vi "RTS MX Data.vi"(8 "Error In":errorcluster, 10 "Station":u8, 11 "Chamber 1 Data in":T1 {"Room PID Settings"."Room Dehumid Temperature I (*RM Dehum I1)" max=30000 step=1; "Room PID Settings"."Room Dehumid Temperature P (*RM Dehum P1)" max=30000 step=1; "Room PID Settings"."Room Cool Temperature I (*RM Cool I1)" max=30000 step=1; "Room PID Settings"."Room Cool Temperature P (*RM Cool P1)" max=30000 step=1; "Room PID Settings"."Room Heat I (*RM Heat I1)" max=30000 step=1; "Room PID Settings"."Room Heat P (*RM Heat P1)" max=30000 step=1; "Room PID Settings"."Room Humidity I (*RM Hum I1)" max=30000 step=1; "Room PID Settings"."Room Humidity P (*RM Hum P1)" max=30000 step=1; "Room PID Settings"."Room Dry I (*RM Dry I1)" max=30000 step=1; "Room PID Settings"."Room Dry P(*RM Dry P1)" max=30000 step=1; "Station 8"."Voltage (V):Element 1 Avg" format="%.3g"; "Station 8"."Voltage (V):Element 2 Avg" format="%.3g"; "Station 8"."Max Watt Hours" format="%.3g"; "Station 8"."Power Factor:Element 2" format="%.3g"; "Station 8"."Power Factor:Element 1" format="%.3g"; "Station 8"."Apparent Power (VA):Element 2" format="%.3g"; "Station 8"."Apparent Power (VA):Element 1" format="%.3g"; "Station 8"."Frequency (Hz):Element 1" format="%.3g"; "Station 8"."Time:Element 1" format="%.3g"; "Station 8"."Voltage Crest Factor:Element 2" format="%.3g"; "Station 8"."Voltage Crest Factor:Element 1" format="%.3g"; "Station 8"."Voltage Harmonic (%):Element 2" format="%.3g"; "Station 8"."Voltage Harmonic (%):Element 1" format="%.3g"; "Station 8"."Current Crest Factor:Element 2" format="%.3g"; "Station 8"."Current Crest Factor:Element 1" format="%.3g"; "Station 8"."Voltage (V):Element 1" format="%.3g"; "Station 8"."Voltage (V):Element 2" format="%.3g"; "Station 8"."Watt Hours (Wh):Sigma" format="%.3f"; "Station 8"."Power (W):Sigma" format="%.3g"; "Station 8"."Current (A):Element 2" format="%.3g"; "Station 8"."Current (A):Element 1" format="%.3g"; "Station 7"."Voltage (V):Element 1 Avg" format="%.3g"; "Station 7"."Voltage (V):Element 2 Avg" format="%.3g"; "Station 7"."Max Watt Hours" format="%.3g"; "Station 7"."Power Factor:Element 2" format="%.3g"; "Station 7"."Power Factor:Element 1" format="%.3g"; "Station 7"."Apparent Power (VA):Element 2" format="%.3g"; "Station 7"."Apparent Power (VA):Element 1" format="%.3g"; "Station 7"."Frequency (Hz):Element 1" format="%.3g"; "Station 7"."Time:Element 1" format="%.3g"; "Station 7"."Voltage Crest Factor:Element 2" format="%.3g"; "Station 7"."Voltage Crest Factor:Element 1" format="%.3g"; "Station 7"."Voltage Harmonic (%):Element 2" format="%.3g"; "Station 7"."Voltage Harmonic (%):Element 1" format="%.3g"; "Station 7"."Current Crest Factor:Element 2" format="%.3g"; "Station 7"."Current Crest Factor:Element 1" format="%.3g"; "Station 7"."Voltage (V):Element 1" format="%.3g"; "Station 7"."Voltage (V):Element 2" format="%.3g"; "Station 7"."Watt Hours (Wh):Sigma" format="%.3f"; "Station 7"."Power (W):Sigma" format="%.3g"; "Station 7"."Current (A):Element 2" format="%.3g"; "Station 7"."Current (A):Element 1" format="%.3g"; "Station 6"."Voltage (V):Element 1 Avg" format="%.3g"; "Station 6"."Voltage (V):Element 2 Avg" format="%.3g"; "Station 6"."Max Watt Hours" format="%.3g"; "Station 6"."Power Factor:Element 2" format="%.3g"; "Station 6"."Power Factor:Element 1" format="%.3g"; "Station 6"."Apparent Power (VA):Element 2" format="%.3g"; "Station 6"."Apparent Power (VA):Element 1" format="%.3g"; "Station 6"."Frequency (Hz):Element 1" format="%.3g"; "Station 6"."Time:Element 1" format="%.3g"; "Station 6"."Voltage Crest Factor:Element 2" format="%.3g"; "Station 6"."Voltage Crest Factor:Element 1" format="%.3g"; "Station 6"."Voltage Harmonic (%):Element 2" format="%.3g"; "Station 6"."Voltage Harmonic (%):Element 1" format="%.3g"; "Station 6"."Current Crest Factor:Element 2" format="%.3g"; "Station 6"."Current Crest Factor:Element 1" format="%.3g"; "Station 6"."Voltage (V):Element 1" format="%.3g"; "Station 6"."Voltage (V):Element 2" format="%.3g"; "Station 6"."Watt Hours (Wh):Sigma" format="%.3f"; "Station 6"."Power (W):Sigma" format="%.3g"; "Station 6"."Current (A):Element 2" format="%.3g"; "Station 6"."Current (A):Element 1" format="%.3g"; "Station 5"."Voltage (V):Element 1 Avg" format="%.3g"; "Station 5"."Voltage (V):Element 2 Avg" format="%.3g"; "Station 5"."Max Watt Hours" format="%.3g"; "Station 5"."Power Factor:Element 2" format="%.3g"; "Station 5"."Power Factor:Element 1" format="%.3g"; "Station 5"."Apparent Power (VA):Element 2" format="%.3g"; "Station 5"."Apparent Power (VA):Element 1" format="%.3g"; "Station 5"."Frequency (Hz):Element 1" format="%.3g"; "Station 5"."Time:Element 1" format="%.3g"; "Station 5"."Voltage Crest Factor:Element 2" format="%.3g"; "Station 5"."Voltage Crest Factor:Element 1" format="%.3g"; "Station 5"."Voltage Harmonic (%):Element 2" format="%.3g"; "Station 5"."Voltage Harmonic (%):Element 1" format="%.3g"; "Station 5"."Current Crest Factor:Element 2" format="%.3g"; "Station 5"."Current Crest Factor:Element 1" format="%.3g"; "Station 5"."Voltage (V):Element 1" format="%.3g"; "Station 5"."Voltage (V):Element 2" format="%.3g"; "Station 5"."Watt Hours (Wh):Sigma" format="%.3f"; "Station 5"."Power (W):Sigma" format="%.3g"; "Station 5"."Current (A):Element 2" format="%.3g"; "Station 5"."Current (A):Element 1" format="%.3g"; "Station 4"."Voltage (V):Element 1 Avg" format="%.3g"; "Station 4"."Voltage (V):Element 2 Avg" format="%.3g"; "Station 4"."Max Watt Hours" format="%.3g"; "Station 4"."Power Factor:Element 2" format="%.3g"; "Station 4"."Power Factor:Element 1" format="%.3g"; "Station 4"."Apparent Power (VA):Element 2" format="%.3g"; "Station 4"."Apparent Power (VA):Element 1" format="%.3g"; "Station 4"."Frequency (Hz):Element 1" format="%.3g"; "Station 4"."Time:Element 1" format="%.3g"; "Station 4"."Voltage Crest Factor:Element 2" format="%.3g"; "Station 4"."Voltage Crest Factor:Element 1" format="%.3g"; "Station 4"."Voltage Harmonic (%):Element 2" format="%.3g"; "Station 4"."Voltage Harmonic (%):Element 1" format="%.3g"; "Station 4"."Current Crest Factor:Element 2" format="%.3g"; "Station 4"."Current Crest Factor:Element 1" format="%.3g"; "Station 4"."Voltage (V):Element 1" format="%.3g"; "Station 4"."Voltage (V):Element 2" format="%.3g"; "Station 4"."Watt Hours (Wh):Sigma" format="%.3f"; "Station 4"."Power (W):Sigma" format="%.3g"; "Station 4"."Current (A):Element 2" format="%.3g"; "Station 4"."Current (A):Element 1" format="%.3g"; "Station 3"."Voltage (V):Element 1 Avg" format="%.3g"; "Station 3"."Voltage (V):Element 2 Avg" format="%.3g"; "Station 3"."Max Watt Hours" format="%.3g"; "Station 3"."Power Factor:Element 2" format="%.3g"; "Station 3"."Power Factor:Element 1" format="%.3g"; "Station 3"."Apparent Power (VA):Element 2" format="%.3g"; "Station 3"."Apparent Power (VA):Element 1" format="%.3g"; "Station 3"."Frequency (Hz):Element 1" format="%.3g"; "Station 3"."Time:Element 1" format="%.3g"; "Station 3"."Voltage Crest Factor:Element 2" format="%.3g"; "Station 3"."Voltage Crest Factor:Element 1" format="%.3g"; "Station 3"."Voltage Harmonic (%):Element 2" format="%.3g"; "Station 3"."Voltage Harmonic (%):Element 1" format="%.3g"; "Station 3"."Current Crest Factor:Element 2" format="%.3g"; "Station 3"."Current Crest Factor:Element 1" format="%.3g"; "Station 3"."Voltage (V):Element 1" format="%.3g"; "Station 3"."Voltage (V):Element 2" format="%.3g"; "Station 3"."Watt Hours (Wh):Sigma" format="%.3f"; "Station 3"."Power (W):Sigma" format="%.3g"; "Station 3"."Current (A):Element 2" format="%.3g"; "Station 3"."Current (A):Element 1" format="%.3g"; "Station 2"."Voltage (V):Element 1 Avg" format="%.3g"; "Station 2"."Voltage (V):Element 2 Avg" format="%.3g"; "Station 2"."Max Watt Hours" format="%.3g"; "Station 2"."Power Factor:Element 2" format="%.3g"; "Station 2"."Power Factor:Element 1" format="%.3g"; "Station 2"."Apparent Power (VA):Element 2" format="%.3g"; "Station 2"."Apparent Power (VA):Element 1" format="%.3g"; "Station 2"."Frequency (Hz):Element 1" format="%.3g"; "Station 2"."Time:Element 1" format="%.3g"; "Station 2"."Voltage Crest Factor:Element 2" format="%.3g"; "Station 2"."Voltage Crest Factor:Element 1" format="%.3g"; "Station 2"."Voltage Harmonic (%):Element 2" format="%.3g"; "Station 2"."Voltage Harmonic (%):Element 1" format="%.3g"; "Station 2"."Current Crest Factor:Element 2" format="%.3g"; "Station 2"."Current Crest Factor:Element 1" format="%.3g"; "Station 2"."Voltage (V):Element 1" format="%.3g"; "Station 2"."Voltage (V):Element 2" format="%.3g"; "Station 2"."Watt Hours (Wh):Sigma" format="%.3f"; "Station 2"."Power (W):Sigma" format="%.3g"; "Station 2"."Current (A):Element 2" format="%.3g"; "Station 2"."Current (A):Element 1" format="%.3g"; "Station 1"."Voltage (V):Element 1 Avg" format="%.3g"; "Station 1"."Voltage (V):Element 2 Avg" format="%.3g"; "Station 1"."Max Watt Hours" format="%.3g"; "Station 1"."Power Factor:Element 2" format="%.3g"; "Station 1"."Power Factor:Element 1" format="%.3g"; "Station 1"."Apparent Power (VA):Element 2" format="%.3g"; "Station 1"."Apparent Power (VA):Element 1" format="%.3g"; "Station 1"."Frequency (Hz):Element 1" format="%.3g"; "Station 1"."Time:Element 1" format="%.3g"; "Station 1"."Voltage Crest Factor:Element 2" format="%.3g"; "Station 1"."Voltage Crest Factor:Element 1" format="%.3g"; "Station 1"."Voltage Harmonic (%):Element 2" format="%.3g"; "Station 1"."Voltage Harmonic (%):Element 1" format="%.3g"; "Station 1"."Current Crest Factor:Element 2" format="%.3g"; "Station 1"."Current Crest Factor:Element 1" format="%.3g"; "Station 1"."Voltage (V):Element 1" format="%.3g"; "Station 1"."Voltage (V):Element 2" format="%.3g"; "Station 1"."Watt Hours (Wh):Sigma" format="%.3f"; "Station 1"."Power (W):Sigma" format="%.3g"; "Station 1"."Current (A):Element 2" format="%.3g"; "Station 1"."Current (A):Element 1" format="%.3g"}) -> (0 "Error Out":errorcluster, 1 "Data MX (DBL)":dbl[](array[numeric]), 2 "Data MX":string[][](array[string]), 3 "Chamber 1 Data Out":T1 {"Room PID Settings"."Room Dehumid Temperature I (*RM Dehum I1)" max=30000 step=1; "Room PID Settings"."Room Dehumid Temperature P (*RM Dehum P1)" max=30000 step=1; "Room PID Settings"."Room Cool Temperature I (*RM Cool I1)" max=30000 step=1; "Room PID Settings"."Room Cool Temperature P (*RM Cool P1)" max=30000 step=1; "Room PID Settings"."Room Heat I (*RM Heat I1)" max=30000 step=1; "Room PID Settings"."Room Heat P (*RM Heat P1)" max=30000 step=1; "Room PID Settings"."Room Humidity I (*RM Hum I1)" max=30000 step=1; "Room PID Settings"."Room Humidity P (*RM Hum P1)" max=30000 step=1; "Room PID Settings"."Room Dry I (*RM Dry I1)" max=30000 step=1; "Room PID Settings"."Room Dry P(*RM Dry P1)" max=30000 step=1; "Station 8"."Voltage (V):Element 1 Avg" format="%.3g"; "Station 8"."Voltage (V):Element 2 Avg" format="%.3g"; "Station 8"."Max Watt Hours" format="%.3g"; "Station 8"."Power Factor:Element 2" format="%.3g"; "Station 8"."Power Factor:Element 1" format="%.3g"; "Station 8"."Apparent Power (VA):Element 2" format="%.3g"; "Station 8"."Apparent Power (VA):Element 1" format="%.3g"; "Station 8"."Frequency (Hz):Element 1" format="%.3g"; "Station 8"."Time:Element 1" format="%.3g"; "Station 8"."Voltage Crest Factor:Element 2" format="%.3g"; "Station 8"."Voltage Crest Factor:Element 1" format="%.3g"; "Station 8"."Voltage Harmonic (%):Element 2" format="%.3g"; "Station 8"."Voltage Harmonic (%):Element 1" format="%.3g"; "Station 8"."Current Crest Factor:Element 2" format="%.3g"; "Station 8"."Current Crest Factor:Element 1" format="%.3g"; "Station 8"."Voltage (V):Element 1" format="%.3g"; "Station 8"."Voltage (V):Element 2" format="%.3g"; "Station 8"."Watt Hours (Wh):Sigma" format="%.3f"; "Station 8"."Power (W):Sigma" format="%.3g"; "Station 8"."Current (A):Element 2" format="%.3g"; "Station 8"."Current (A):Element 1" format="%.3g"; "Station 7"."Voltage (V):Element 1 Avg" format="%.3g"; "Station 7"."Voltage (V):Element 2 Avg" format="%.3g"; "Station 7"."Max Watt Hours" format="%.3g"; "Station 7"."Power Factor:Element 2" format="%.3g"; "Station 7"."Power Factor:Element 1" format="%.3g"; "Station 7"."Apparent Power (VA):Element 2" format="%.3g"; "Station 7"."Apparent Power (VA):Element 1" format="%.3g"; "Station 7"."Frequency (Hz):Element 1" format="%.3g"; "Station 7"."Time:Element 1" format="%.3g"; "Station 7"."Voltage Crest Factor:Element 2" format="%.3g"; "Station 7"."Voltage Crest Factor:Element 1" format="%.3g"; "Station 7"."Voltage Harmonic (%):Element 2" format="%.3g"; "Station 7"."Voltage Harmonic (%):Element 1" format="%.3g"; "Station 7"."Current Crest Factor:Element 2" format="%.3g"; "Station 7"."Current Crest Factor:Element 1" format="%.3g"; "Station 7"."Voltage (V):Element 1" format="%.3g"; "Station 7"."Voltage (V):Element 2" format="%.3g"; "Station 7"."Watt Hours (Wh):Sigma" format="%.3f"; "Station 7"."Power (W):Sigma" format="%.3g"; "Station 7"."Current (A):Element 2" format="%.3g"; "Station 7"."Current (A):Element 1" format="%.3g"; "Station 6"."Voltage (V):Element 1 Avg" format="%.3g"; "Station 6"."Voltage (V):Element 2 Avg" format="%.3g"; "Station 6"."Max Watt Hours" format="%.3g"; "Station 6"."Power Factor:Element 2" format="%.3g"; "Station 6"."Power Factor:Element 1" format="%.3g"; "Station 6"."Apparent Power (VA):Element 2" format="%.3g"; "Station 6"."Apparent Power (VA):Element 1" format="%.3g"; "Station 6"."Frequency (Hz):Element 1" format="%.3g"; "Station 6"."Time:Element 1" format="%.3g"; "Station 6"."Voltage Crest Factor:Element 2" format="%.3g"; "Station 6"."Voltage Crest Factor:Element 1" format="%.3g"; "Station 6"."Voltage Harmonic (%):Element 2" format="%.3g"; "Station 6"."Voltage Harmonic (%):Element 1" format="%.3g"; "Station 6"."Current Crest Factor:Element 2" format="%.3g"; "Station 6"."Current Crest Factor:Element 1" format="%.3g"; "Station 6"."Voltage (V):Element 1" format="%.3g"; "Station 6"."Voltage (V):Element 2" format="%.3g"; "Station 6"."Watt Hours (Wh):Sigma" format="%.3f"; "Station 6"."Power (W):Sigma" format="%.3g"; "Station 6"."Current (A):Element 2" format="%.3g"; "Station 6"."Current (A):Element 1" format="%.3g"; "Station 5"."Voltage (V):Element 1 Avg" format="%.3g"; "Station 5"."Voltage (V):Element 2 Avg" format="%.3g"; "Station 5"."Max Watt Hours" format="%.3g"; "Station 5"."Power Factor:Element 2" format="%.3g"; "Station 5"."Power Factor:Element 1" format="%.3g"; "Station 5"."Apparent Power (VA):Element 2" format="%.3g"; "Station 5"."Apparent Power (VA):Element 1" format="%.3g"; "Station 5"."Frequency (Hz):Element 1" format="%.3g"; "Station 5"."Time:Element 1" format="%.3g"; "Station 5"."Voltage Crest Factor:Element 2" format="%.3g"; "Station 5"."Voltage Crest Factor:Element 1" format="%.3g"; "Station 5"."Voltage Harmonic (%):Element 2" format="%.3g"; "Station 5"."Voltage Harmonic (%):Element 1" format="%.3g"; "Station 5"."Current Crest Factor:Element 2" format="%.3g"; "Station 5"."Current Crest Factor:Element 1" format="%.3g"; "Station 5"."Voltage (V):Element 1" format="%.3g"; "Station 5"."Voltage (V):Element 2" format="%.3g"; "Station 5"."Watt Hours (Wh):Sigma" format="%.3f"; "Station 5"."Power (W):Sigma" format="%.3g"; "Station 5"."Current (A):Element 2" format="%.3g"; "Station 5"."Current (A):Element 1" format="%.3g"; "Station 4"."Voltage (V):Element 1 Avg" format="%.3g"; "Station 4"."Voltage (V):Element 2 Avg" format="%.3g"; "Station 4"."Max Watt Hours" format="%.3g"; "Station 4"."Power Factor:Element 2" format="%.3g"; "Station 4"."Power Factor:Element 1" format="%.3g"; "Station 4"."Apparent Power (VA):Element 2" format="%.3g"; "Station 4"."Apparent Power (VA):Element 1" format="%.3g"; "Station 4"."Frequency (Hz):Element 1" format="%.3g"; "Station 4"."Time:Element 1" format="%.3g"; "Station 4"."Voltage Crest Factor:Element 2" format="%.3g"; "Station 4"."Voltage Crest Factor:Element 1" format="%.3g"; "Station 4"."Voltage Harmonic (%):Element 2" format="%.3g"; "Station 4"."Voltage Harmonic (%):Element 1" format="%.3g"; "Station 4"."Current Crest Factor:Element 2" format="%.3g"; "Station 4"."Current Crest Factor:Element 1" format="%.3g"; "Station 4"."Voltage (V):Element 1" format="%.3g"; "Station 4"."Voltage (V):Element 2" format="%.3g"; "Station 4"."Watt Hours (Wh):Sigma" format="%.3f"; "Station 4"."Power (W):Sigma" format="%.3g"; "Station 4"."Current (A):Element 2" format="%.3g"; "Station 4"."Current (A):Element 1" format="%.3g"; "Station 3"."Voltage (V):Element 1 Avg" format="%.3g"; "Station 3"."Voltage (V):Element 2 Avg" format="%.3g"; "Station 3"."Max Watt Hours" format="%.3g"; "Station 3"."Power Factor:Element 2" format="%.3g"; "Station 3"."Power Factor:Element 1" format="%.3g"; "Station 3"."Apparent Power (VA):Element 2" format="%.3g"; "Station 3"."Apparent Power (VA):Element 1" format="%.3g"; "Station 3"."Frequency (Hz):Element 1" format="%.3g"; "Station 3"."Time:Element 1" format="%.3g"; "Station 3"."Voltage Crest Factor:Element 2" format="%.3g"; "Station 3"."Voltage Crest Factor:Element 1" format="%.3g"; "Station 3"."Voltage Harmonic (%):Element 2" format="%.3g"; "Station 3"."Voltage Harmonic (%):Element 1" format="%.3g"; "Station 3"."Current Crest Factor:Element 2" format="%.3g"; "Station 3"."Current Crest Factor:Element 1" format="%.3g"; "Station 3"."Voltage (V):Element 1" format="%.3g"; "Station 3"."Voltage (V):Element 2" format="%.3g"; "Station 3"."Watt Hours (Wh):Sigma" format="%.3f"; "Station 3"."Power (W):Sigma" format="%.3g"; "Station 3"."Current (A):Element 2" format="%.3g"; "Station 3"."Current (A):Element 1" format="%.3g"; "Station 2"."Voltage (V):Element 1 Avg" format="%.3g"; "Station 2"."Voltage (V):Element 2 Avg" format="%.3g"; "Station 2"."Max Watt Hours" format="%.3g"; "Station 2"."Power Factor:Element 2" format="%.3g"; "Station 2"."Power Factor:Element 1" format="%.3g"; "Station 2"."Apparent Power (VA):Element 2" format="%.3g"; "Station 2"."Apparent Power (VA):Element 1" format="%.3g"; "Station 2"."Frequency (Hz):Element 1" format="%.3g"; "Station 2"."Time:Element 1" format="%.3g"; "Station 2"."Voltage Crest Factor:Element 2" format="%.3g"; "Station 2"."Voltage Crest Factor:Element 1" format="%.3g"; "Station 2"."Voltage Harmonic (%):Element 2" format="%.3g"; "Station 2"."Voltage Harmonic (%):Element 1" format="%.3g"; "Station 2"."Current Crest Factor:Element 2" format="%.3g"; "Station 2"."Current Crest Factor:Element 1" format="%.3g"; "Station 2"."Voltage (V):Element 1" format="%.3g"; "Station 2"."Voltage (V):Element 2" format="%.3g"; "Station 2"."Watt Hours (Wh):Sigma" format="%.3f"; "Station 2"."Power (W):Sigma" format="%.3g"; "Station 2"."Current (A):Element 2" format="%.3g"; "Station 2"."Current (A):Element 1" format="%.3g"; "Station 1"."Voltage (V):Element 1 Avg" format="%.3g"; "Station 1"."Voltage (V):Element 2 Avg" format="%.3g"; "Station 1"."Max Watt Hours" format="%.3g"; "Station 1"."Power Factor:Element 2" format="%.3g"; "Station 1"."Power Factor:Element 1" format="%.3g"; "Station 1"."Apparent Power (VA):Element 2" format="%.3g"; "Station 1"."Apparent Power (VA):Element 1" format="%.3g"; "Station 1"."Frequency (Hz):Element 1" format="%.3g"; "Station 1"."Time:Element 1" format="%.3g"; "Station 1"."Voltage Crest Factor:Element 2" format="%.3g"; "Station 1"."Voltage Crest Factor:Element 1" format="%.3g"; "Station 1"."Voltage Harmonic (%):Element 2" format="%.3g"; "Station 1"."Voltage Harmonic (%):Element 1" format="%.3g"; "Station 1"."Current Crest Factor:Element 2" format="%.3g"; "Station 1"."Current Crest Factor:Element 1" format="%.3g"; "Station 1"."Voltage (V):Element 1" format="%.3g"; "Station 1"."Voltage (V):Element 2" format="%.3g"; "Station 1"."Watt Hours (Wh):Sigma" format="%.3f"; "Station 1"."Power (W):Sigma" format="%.3g"; "Station 1"."Current (A):Element 2" format="%.3g"; "Station 1"."Current (A):Element 1" format="%.3g"})   [LabVIEW 2016]
uses:
  Type Definitions/RTS Chamber Data.ctl
  Utility/Type Definitions/UTILITY Power Data.ctl
  Type Definitions/RTS Chamber TCs.ctl
  Type Definitions/RTS MX5 AUX Data.ctl
  Drivers/WAGO 750-881/Type Definitions/Wago Door Relays.ctl
  Drivers/WAGO 750-881/Type Definitions/Wago Contactor Settings.ctl
  Drivers/WAGO 750-881/Type Definitions/Wago Ground Leakage.ctl
  Drivers/WAGO 750-881/Type Definitions/Wago Measured Input Data.ctl
  Drivers/WAGO 750-881/Type Definitions/Wago Room Setpoint Targets.ctl
  Drivers/WAGO 750-881/Type Definitions/Wago Room PID Settings.ctl
  Drivers/WAGO 750-881/Type Definitions/Wago Room Condtions.ctl
panel:
  # "APLUS"
  # "MX100"
  # "Wago Controller"
  # "APLUS"
  # "MX100"
  # "Wago Controller"
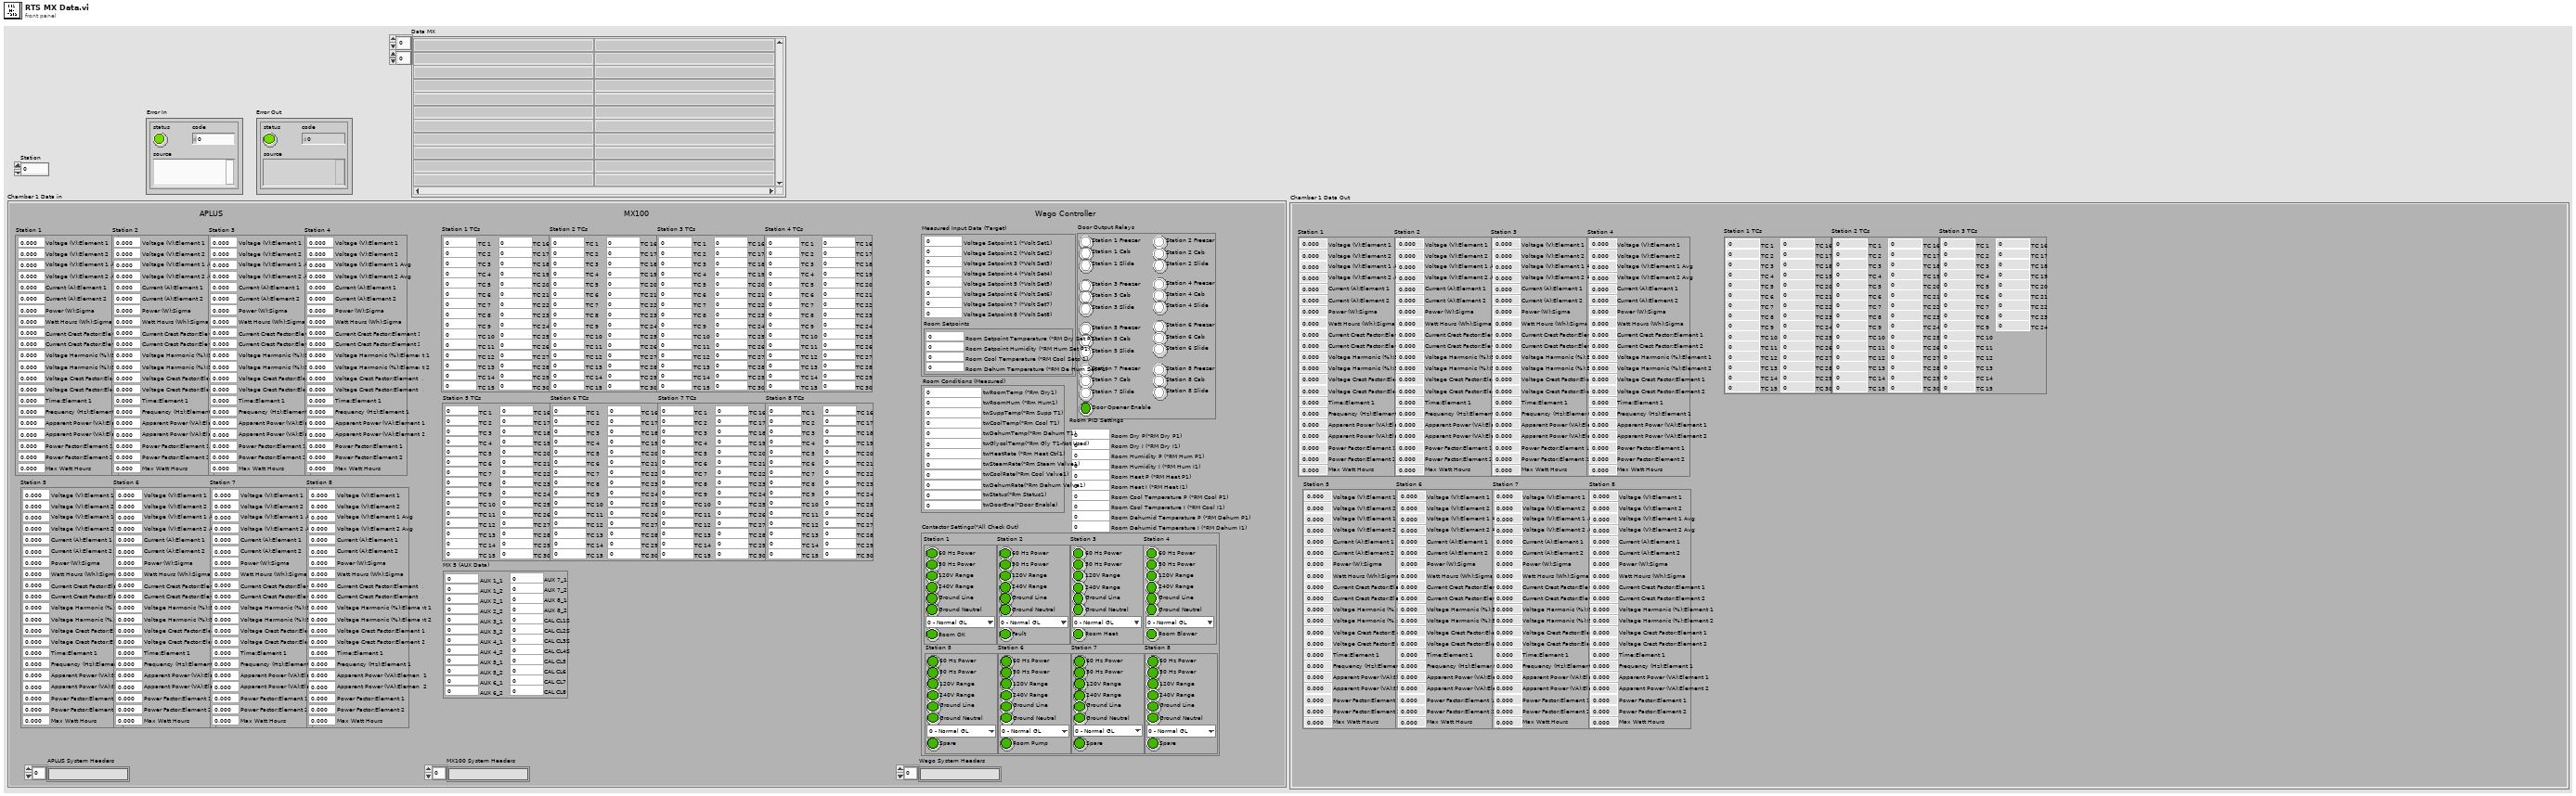
[diagram p1: front panel]
types:
  T1 = typedef "RTS Chamber Data.ctl" = cluster{"Station 1":T2, "Station 2":T2, "Station 3":T2, "Station 4":T2, "Station 5":T2, "Station 6":T2, "Station 7":T2, "Station 8":T2, "Station 1 TCs":T3, "Station 2 TCs":T3, "Station 3 TCs":T3, "Station 4 TCs":T3, "Station 5 TCs":T3, "Station 6 TCs":T3, "Station 7 TCs":T3, "Station 8 TCs":T3, "MX 5 (AUX Data)":T4, "Door Output Relays":T5, "Contactor Settings(*All Check Out)":T6, "Measured Input Data (Target)":T8, "Room PID Settings":T10, "Room Conditions (Measured)":T11, "APLUS System Headers":string[], "MX100 System Headers":string[], "Wago System Headers":string[]}
  T2 = typedef "UTILITY Power Data.ctl" = cluster{"Current (A):Element 1":dbl, "Current (A):Element 2":dbl, "Power (W):Sigma":dbl, "Watt Hours (Wh):Sigma":dbl, "Voltage (V):Element 2":dbl, "Voltage (V):Element 1":dbl, "Current Crest Factor:Element 1":dbl, "Current Crest Factor:Element 2":dbl, "Voltage Harmonic (%):Element 1":dbl, "Voltage Harmonic (%):Element 2":dbl, "Voltage Crest Factor:Element 1":dbl, "Voltage Crest Factor:Element 2":dbl, "Time:Element 1":dbl, "Frequency (Hz):Element 1":dbl, "Apparent Power (VA):Element 1":dbl, "Apparent Power (VA):Element 2":dbl, "Power Factor:Element 1":dbl, "Power Factor:Element 2":dbl, "Max Watt Hours":dbl, "Voltage (V):Element 2 Avg":dbl, "Voltage (V):Element 1 Avg":dbl}
  T3 = typedef "RTS Chamber TCs.ctl" = cluster{"TC 1":dbl, "TC 2":dbl, "TC 3":dbl, "TC 4":dbl, "TC 5":dbl, "TC 6":dbl, "TC 7":dbl, "TC 8":dbl, "TC 9":dbl, "TC 10":dbl, "TC 11":dbl, "TC 12":dbl, "TC 13":dbl, "TC 14":dbl, "TC 15":dbl, "TC 16":dbl, "TC 17":dbl, "TC 18":dbl, "TC 19":dbl, "TC 20":dbl, "TC 21":dbl, "TC 22":dbl, "TC 23":dbl, "TC 24":dbl, "TC 25":dbl, "TC 26":dbl, "TC 27":dbl, "TC 28":dbl, "TC 29":dbl, "TC 30":dbl}
  T4 = typedef "RTS MX5 AUX Data.ctl" = cluster{"AUX 1_1":dbl, "AUX 1_2":dbl, "AUX 2_1":dbl, "AUX 2_2":dbl, "AUX 3_1":dbl, "AUX 3_2":dbl, "AUX 4_1":dbl, "AUX 4_2":dbl, "AUX 5_1":dbl, "AUX 5_2":dbl, "AUX 6_1":dbl, "AUX 6_2":dbl, "AUX 7_1":dbl, "AUX 7_2":dbl, "AUX 8_1":dbl, "AUX 8_2":dbl, "CAL CL1S":dbl, "CAL CL2S":dbl, "CAL CL3S":dbl, "CAL CL4S":dbl, "CAL CL5":dbl, "CAL CL6":dbl, "CAL CL7":dbl, "CAL CL8":dbl}
  T5 = typedef "Wago Door Relays.ctl" = cluster{"Station 1 Freezer":bool, "Station 1 Cab":bool, "Station 1 Slide":bool, "Station 2 Freezer":bool, "Station 2 Cab":bool, "Station 2 Slide":bool, "Station 3 Freezer":bool, "Station 3 Cab":bool, "Station 3 Slide":bool, "Station 4 Freezer":bool, "Station 4 Cab":bool, "Station 4 Slide":bool, "Station 5 Freezer":bool, "Station 5 Cab":bool, "Station 5 Slide":bool, "Station 6 Freezer":bool, "Station 6 Cab":bool, "Station 6 Slide":bool, "Station 7 Freezer":bool, "Station 7 Cab":bool, "Station 7 Slide":bool, "Station 8 Freezer":bool, "Station 8 Cab":bool, "Station 8 Slide":bool, "Door Opener Enable":bool}
  T6 = typedef "Wago Contactor Settings.ctl" = cluster{"Station 1":cluster{"60 Hz Power":bool, "50 Hz Power":bool, "120V Range":bool, "240V Range":bool, "Ground Line":bool, "Ground Neutral":bool, "Room OK":bool, "Ground Leakage":T7}, "Station 2":cluster{"60 Hz Power":bool, "50 Hz Power":bool, "120V Range":bool, "240V Range":bool, "Ground Line":bool, "Ground Neutral":bool, "Fault":bool, "Ground Leakage":T7}, "Station 3":cluster{"60 Hz Power":bool, "50 Hz Power":bool, "120V Range":bool, "240V Range":bool, "Ground Line":bool, "Ground Neutral":bool, "Room Heat":bool, "Ground Leakage":T7}, "Station 4":cluster{"60 Hz Power":bool, "50 Hz Power":bool, "120V Range":bool, "240V Range":bool, "Ground Line":bool, "Ground Neutral":bool, "Room Blower":bool, "Ground Leakage":T7}, "Station 5":cluster{"60 Hz Power":bool, "50 Hz Power":bool, "120V Range":bool, "240V Range":bool, "Ground Line":bool, "Ground Neutral":bool, "Spare":bool, "Ground Leakage":T7}, "Station 6":cluster{"60 Hz Power":bool, "50 Hz Power":bool, "120V Range":bool, "240V Range":bool, "Ground Line":bool, "Ground Neutral":bool, "Room Pump":bool, "Ground Leakage":T7}, "Station 7":cluster{"60 Hz Power":bool, "50 Hz Power":bool, "120V Range":bool, "240V Range":bool, "Ground Line":bool, "Ground Neutral":bool, "Spare":bool, "Ground Leakage":T7}, "Station 8":cluster{"60 Hz Power":bool, "50 Hz Power":bool, "120V Range":bool, "240V Range":bool, "Ground Line":bool, "Ground Neutral":bool, "Spare":bool, "Ground Leakage":T7}}
  T7 = typedef "Wago Ground Leakage.ctl" = enum16{"0 - Normal GL", "1 - Measure GL"}
  T8 = typedef "Wago Measured Input Data.ctl" = cluster{"Voltage Setpoint 1 (*Volt Set1)":dbl, "Voltage Setpoint 2 (*Volt Set2)":dbl, "Voltage Setpoint 3 (*Volt Set3)":dbl, "Voltage Setpoint 4 (*Volt Set4)":dbl, "Voltage Setpoint 5 (*Volt Set5)":dbl, "Voltage Setpoint 6 (*Volt Set6)":dbl, "Voltage Setpoint 7 (*Volt Set7)":dbl, "Voltage Setpoint 8 (*Volt Set8)":dbl, "Room Setpoints":T9}
  T9 = typedef "Wago Room Setpoint Targets.ctl" = cluster{"Room Setpoint Temperature (*RM Dry Set P1)":dbl, "Room Setpoint Humidity (*RM Hum Set P1)":dbl, "Room Cool Temperature (*RM Cool Setp 1)":dbl, "Room Dehum Temperature (*RM De Hum Set P1)":dbl}
  T10 = typedef "Wago Room PID Settings.ctl" = cluster{"Room Dry P(*RM Dry P1)":u16, "Room Dry I (*RM Dry I1)":u16, "Room Humidity P (*RM Hum P1)":u16, "Room Humidity I (*RM Hum I1)":u16, "Room Heat P (*RM Heat P1)":u16, "Room Heat I (*RM Heat I1)":u16, "Room Cool Temperature P (*RM Cool P1)":u16, "Room Cool Temperature I (*RM Cool I1)":u16, "Room Dehumid Temperature P (*RM Dehum P1)":u16, "Room Dehumid Temperature I (*RM Dehum I1)":u16}
  T11 = typedef "Wago Room Condtions.ctl" = cluster{"twDoorEna(*Door Enable)":u16, "twStatus(*Rm Status1)":u16, "twRoomTemp (*Rm Dry1)":dbl, "twRoomHum (*Rm Hum1)":dbl, "twSuppTemp(*Rm Supp T1)":dbl, "twCoolTemp(*Rm Cool T1)":dbl, "twDehumTemp(*Rm Dehum T1)":dbl, "twGlycolTemp(*Rm Gly T1-Not Used)":dbl, "twDehumRate(*Rm Dehum Valve1)":dbl, "twCoolRate(*Rm Cool Valve1)":dbl, "twSteamRate(*Rm Steam Valve1)":dbl, "twHeatRate (*Rm Heat Ctrl1)":dbl}
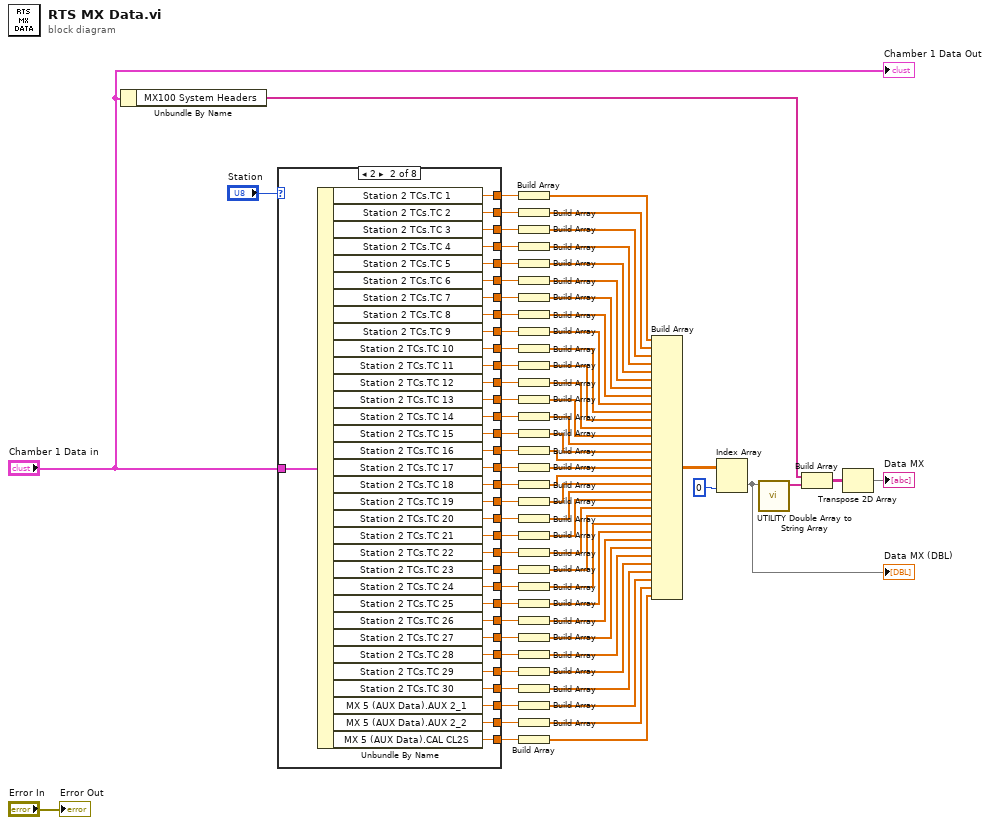
[diagram p0: block diagram]
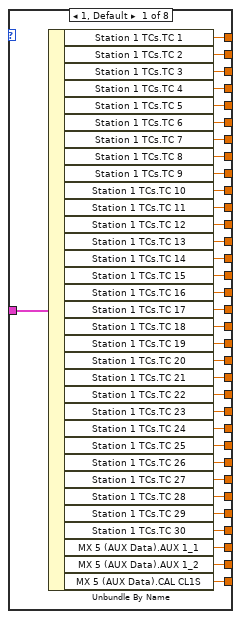
[diagram p2: hidden frame]
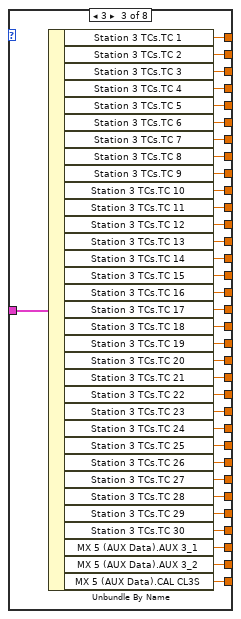
[diagram p3: hidden frame]
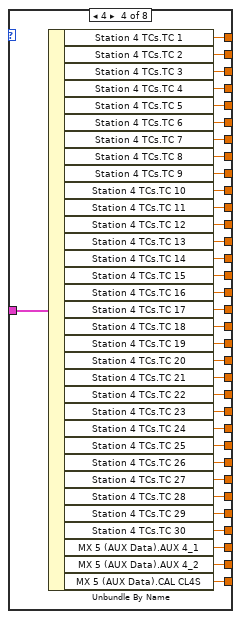
[diagram p4: hidden frame]
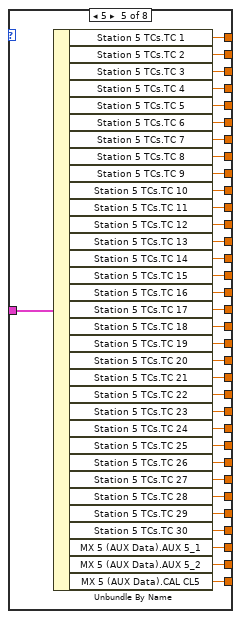
[diagram p5: hidden frame]
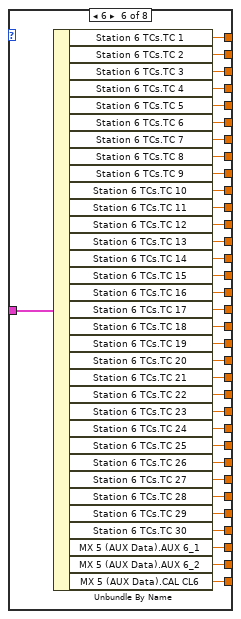
[diagram p6: hidden frame]
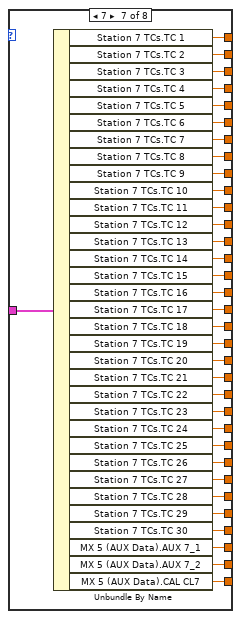
[diagram p7: hidden frame]
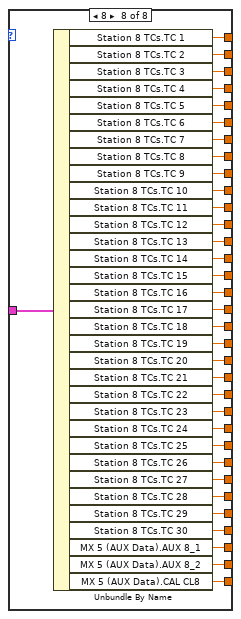
[diagram p8: hidden frame]
diagram:
  n1 = Unbundle By Name("Chamber 1 Data in") -> ("MX100 System Headers"=w38:string[])
  n2 = case shown="2" "Station" {
    tunnel: "Chamber 1 Data in" -> [w110 w144 w178 w212 w246 w280 w314 w348]
    tunnel: [w109 w143 w177 w211 w245 w279 w313 w347] -> w44
    tunnel: [w108 w142 w176 w210 w244 w278 w312 w346] -> w45
    tunnel: [w107 w141 w175 w209 w243 w277 w311 w345] -> w46
    tunnel: [w106 w140 w174 w208 w242 w276 w310 w344] -> w47
    tunnel: [w105 w139 w173 w207 w241 w275 w309 w343] -> w48
    tunnel: [w104 w138 w172 w206 w240 w274 w308 w342] -> w49
    tunnel: [w103 w137 w171 w205 w239 w273 w307 w341] -> w50
    tunnel: [w102 w136 w170 w204 w238 w272 w306 w340] -> w51
    tunnel: [w101 w135 w169 w203 w237 w271 w305 w339] -> w52
    tunnel: [w100 w134 w168 w202 w236 w270 w304 w338] -> w53
    tunnel: [w99 w133 w167 w201 w235 w269 w303 w337] -> w54
    tunnel: [w98 w132 w166 w200 w234 w268 w302 w336] -> w55
    tunnel: [w97 w131 w165 w199 w233 w267 w301 w335] -> w56
    tunnel: [w96 w130 w164 w198 w232 w266 w300 w334] -> w57
    tunnel: [w95 w129 w163 w197 w231 w265 w299 w333] -> w58
    tunnel: [w94 w128 w162 w196 w230 w264 w298 w332] -> w59
    tunnel: [w93 w127 w161 w195 w229 w263 w297 w331] -> w60
    tunnel: [w92 w126 w160 w194 w228 w262 w296 w330] -> w61
    tunnel: [w91 w125 w159 w193 w227 w261 w295 w329] -> w62
    tunnel: [w90 w124 w158 w192 w226 w260 w294 w328] -> w63
    tunnel: [w89 w123 w157 w191 w225 w259 w293 w327] -> w64
    tunnel: [w88 w122 w156 w190 w224 w258 w292 w326] -> w65
    tunnel: [w87 w121 w155 w189 w223 w257 w291 w325] -> w66
    tunnel: [w86 w120 w154 w188 w222 w256 w290 w324] -> w67
    tunnel: [w85 w119 w153 w187 w221 w255 w289 w323] -> w68
    tunnel: [w84 w118 w152 w186 w220 w254 w288 w322] -> w69
    tunnel: [w83 w117 w151 w185 w219 w253 w287 w321] -> w70
    tunnel: [w82 w116 w150 w184 w218 w252 w286 w320] -> w71
    tunnel: [w81 w115 w149 w183 w217 w251 w285 w319] -> w72
    tunnel: [w80 w114 w148 w182 w216 w250 w284 w318] -> w73
    tunnel: [w79 w113 w147 w181 w215 w249 w283 w317] -> w74
    tunnel: [w78 w112 w146 w180 w214 w248 w282 w316] -> w75
    tunnel: [w77 w111 w145 w179 w213 w247 w281 w315] -> w76
    frame 1, Default {
      n3 = Unbundle By Name(w110) -> ("Station 1 TCs.TC 1"=w109:dbl, "Station 1 TCs.TC 2"=w108:dbl, "Station 1 TCs.TC 3"=w107:dbl, "Station 1 TCs.TC 4"=w106:dbl, "Station 1 TCs.TC 5"=w105:dbl, "Station 1 TCs.TC 6"=w104:dbl, "Station 1 TCs.TC 7"=w103:dbl, "Station 1 TCs.TC 8"=w102:dbl, "Station 1 TCs.TC 9"=w101:dbl, "Station 1 TCs.TC 10"=w100:dbl, "Station 1 TCs.TC 11"=w99:dbl, "Station 1 TCs.TC 12"=w98:dbl, "Station 1 TCs.TC 13"=w97:dbl, "Station 1 TCs.TC 14"=w96:dbl, "Station 1 TCs.TC 15"=w95:dbl, "Station 1 TCs.TC 16"=w94:dbl, "Station 1 TCs.TC 17"=w93:dbl, "Station 1 TCs.TC 18"=w92:dbl, "Station 1 TCs.TC 19"=w91:dbl, "Station 1 TCs.TC 20"=w90:dbl, "Station 1 TCs.TC 21"=w89:dbl, "Station 1 TCs.TC 22"=w88:dbl, "Station 1 TCs.TC 23"=w87:dbl, "Station 1 TCs.TC 24"=w86:dbl, "Station 1 TCs.TC 25"=w85:dbl, "Station 1 TCs.TC 26"=w84:dbl, "Station 1 TCs.TC 27"=w83:dbl, "Station 1 TCs.TC 28"=w82:dbl, "Station 1 TCs.TC 29"=w81:dbl, "Station 1 TCs.TC 30"=w80:dbl, "MX 5 (AUX Data).AUX 1_1"=w79:dbl, "MX 5 (AUX Data).AUX 1_2"=w78:dbl, "MX 5 (AUX Data).CAL CL1S"=w77:dbl)
    }
    frame 2 {
      n4 = Unbundle By Name(w144) -> ("Station 2 TCs.TC 1"=w143:dbl, "Station 2 TCs.TC 2"=w142:dbl, "Station 2 TCs.TC 3"=w141:dbl, "Station 2 TCs.TC 4"=w140:dbl, "Station 2 TCs.TC 5"=w139:dbl, "Station 2 TCs.TC 6"=w138:dbl, "Station 2 TCs.TC 7"=w137:dbl, "Station 2 TCs.TC 8"=w136:dbl, "Station 2 TCs.TC 9"=w135:dbl, "Station 2 TCs.TC 10"=w134:dbl, "Station 2 TCs.TC 11"=w133:dbl, "Station 2 TCs.TC 12"=w132:dbl, "Station 2 TCs.TC 13"=w131:dbl, "Station 2 TCs.TC 14"=w130:dbl, "Station 2 TCs.TC 15"=w129:dbl, "Station 2 TCs.TC 16"=w128:dbl, "Station 2 TCs.TC 17"=w127:dbl, "Station 2 TCs.TC 18"=w126:dbl, "Station 2 TCs.TC 19"=w125:dbl, "Station 2 TCs.TC 20"=w124:dbl, "Station 2 TCs.TC 21"=w123:dbl, "Station 2 TCs.TC 22"=w122:dbl, "Station 2 TCs.TC 23"=w121:dbl, "Station 2 TCs.TC 24"=w120:dbl, "Station 2 TCs.TC 25"=w119:dbl, "Station 2 TCs.TC 26"=w118:dbl, "Station 2 TCs.TC 27"=w117:dbl, "Station 2 TCs.TC 28"=w116:dbl, "Station 2 TCs.TC 29"=w115:dbl, "Station 2 TCs.TC 30"=w114:dbl, "MX 5 (AUX Data).AUX 2_1"=w113:dbl, "MX 5 (AUX Data).AUX 2_2"=w112:dbl, "MX 5 (AUX Data).CAL CL2S"=w111:dbl)
    }
    frame 3 {
      n5 = Unbundle By Name(w178) -> ("Station 3 TCs.TC 1"=w177:dbl, "Station 3 TCs.TC 2"=w176:dbl, "Station 3 TCs.TC 3"=w175:dbl, "Station 3 TCs.TC 4"=w174:dbl, "Station 3 TCs.TC 5"=w173:dbl, "Station 3 TCs.TC 6"=w172:dbl, "Station 3 TCs.TC 7"=w171:dbl, "Station 3 TCs.TC 8"=w170:dbl, "Station 3 TCs.TC 9"=w169:dbl, "Station 3 TCs.TC 10"=w168:dbl, "Station 3 TCs.TC 11"=w167:dbl, "Station 3 TCs.TC 12"=w166:dbl, "Station 3 TCs.TC 13"=w165:dbl, "Station 3 TCs.TC 14"=w164:dbl, "Station 3 TCs.TC 15"=w163:dbl, "Station 3 TCs.TC 16"=w162:dbl, "Station 3 TCs.TC 17"=w161:dbl, "Station 3 TCs.TC 18"=w160:dbl, "Station 3 TCs.TC 19"=w159:dbl, "Station 3 TCs.TC 20"=w158:dbl, "Station 3 TCs.TC 21"=w157:dbl, "Station 3 TCs.TC 22"=w156:dbl, "Station 3 TCs.TC 23"=w155:dbl, "Station 3 TCs.TC 24"=w154:dbl, "Station 3 TCs.TC 25"=w153:dbl, "Station 3 TCs.TC 26"=w152:dbl, "Station 3 TCs.TC 27"=w151:dbl, "Station 3 TCs.TC 28"=w150:dbl, "Station 3 TCs.TC 29"=w149:dbl, "Station 3 TCs.TC 30"=w148:dbl, "MX 5 (AUX Data).AUX 3_1"=w147:dbl, "MX 5 (AUX Data).AUX 3_2"=w146:dbl, "MX 5 (AUX Data).CAL CL3S"=w145:dbl)
    }
    frame 4 {
      n6 = Unbundle By Name(w212) -> ("Station 4 TCs.TC 1"=w211:dbl, "Station 4 TCs.TC 2"=w210:dbl, "Station 4 TCs.TC 3"=w209:dbl, "Station 4 TCs.TC 4"=w208:dbl, "Station 4 TCs.TC 5"=w207:dbl, "Station 4 TCs.TC 6"=w206:dbl, "Station 4 TCs.TC 7"=w205:dbl, "Station 4 TCs.TC 8"=w204:dbl, "Station 4 TCs.TC 9"=w203:dbl, "Station 4 TCs.TC 10"=w202:dbl, "Station 4 TCs.TC 11"=w201:dbl, "Station 4 TCs.TC 12"=w200:dbl, "Station 4 TCs.TC 13"=w199:dbl, "Station 4 TCs.TC 14"=w198:dbl, "Station 4 TCs.TC 15"=w197:dbl, "Station 4 TCs.TC 16"=w196:dbl, "Station 4 TCs.TC 17"=w195:dbl, "Station 4 TCs.TC 18"=w194:dbl, "Station 4 TCs.TC 19"=w193:dbl, "Station 4 TCs.TC 20"=w192:dbl, "Station 4 TCs.TC 21"=w191:dbl, "Station 4 TCs.TC 22"=w190:dbl, "Station 4 TCs.TC 23"=w189:dbl, "Station 4 TCs.TC 24"=w188:dbl, "Station 4 TCs.TC 25"=w187:dbl, "Station 4 TCs.TC 26"=w186:dbl, "Station 4 TCs.TC 27"=w185:dbl, "Station 4 TCs.TC 28"=w184:dbl, "Station 4 TCs.TC 29"=w183:dbl, "Station 4 TCs.TC 30"=w182:dbl, "MX 5 (AUX Data).AUX 4_1"=w181:dbl, "MX 5 (AUX Data).AUX 4_2"=w180:dbl, "MX 5 (AUX Data).CAL CL4S"=w179:dbl)
    }
    frame 5 {
      n7 = Unbundle By Name(w246) -> ("Station 5 TCs.TC 1"=w245:dbl, "Station 5 TCs.TC 2"=w244:dbl, "Station 5 TCs.TC 3"=w243:dbl, "Station 5 TCs.TC 4"=w242:dbl, "Station 5 TCs.TC 5"=w241:dbl, "Station 5 TCs.TC 6"=w240:dbl, "Station 5 TCs.TC 7"=w239:dbl, "Station 5 TCs.TC 8"=w238:dbl, "Station 5 TCs.TC 9"=w237:dbl, "Station 5 TCs.TC 10"=w236:dbl, "Station 5 TCs.TC 11"=w235:dbl, "Station 5 TCs.TC 12"=w234:dbl, "Station 5 TCs.TC 13"=w233:dbl, "Station 5 TCs.TC 14"=w232:dbl, "Station 5 TCs.TC 15"=w231:dbl, "Station 5 TCs.TC 16"=w230:dbl, "Station 5 TCs.TC 17"=w229:dbl, "Station 5 TCs.TC 18"=w228:dbl, "Station 5 TCs.TC 19"=w227:dbl, "Station 5 TCs.TC 20"=w226:dbl, "Station 5 TCs.TC 21"=w225:dbl, "Station 5 TCs.TC 22"=w224:dbl, "Station 5 TCs.TC 23"=w223:dbl, "Station 5 TCs.TC 24"=w222:dbl, "Station 5 TCs.TC 25"=w221:dbl, "Station 5 TCs.TC 26"=w220:dbl, "Station 5 TCs.TC 27"=w219:dbl, "Station 5 TCs.TC 28"=w218:dbl, "Station 5 TCs.TC 29"=w217:dbl, "Station 5 TCs.TC 30"=w216:dbl, "MX 5 (AUX Data).AUX 5_1"=w215:dbl, "MX 5 (AUX Data).AUX 5_2"=w214:dbl, "MX 5 (AUX Data).CAL CL5"=w213:dbl)
    }
    frame 6 {
      n8 = Unbundle By Name(w280) -> ("Station 6 TCs.TC 1"=w279:dbl, "Station 6 TCs.TC 2"=w278:dbl, "Station 6 TCs.TC 3"=w277:dbl, "Station 6 TCs.TC 4"=w276:dbl, "Station 6 TCs.TC 5"=w275:dbl, "Station 6 TCs.TC 6"=w274:dbl, "Station 6 TCs.TC 7"=w273:dbl, "Station 6 TCs.TC 8"=w272:dbl, "Station 6 TCs.TC 9"=w271:dbl, "Station 6 TCs.TC 10"=w270:dbl, "Station 6 TCs.TC 11"=w269:dbl, "Station 6 TCs.TC 12"=w268:dbl, "Station 6 TCs.TC 13"=w267:dbl, "Station 6 TCs.TC 14"=w266:dbl, "Station 6 TCs.TC 15"=w265:dbl, "Station 6 TCs.TC 16"=w264:dbl, "Station 6 TCs.TC 17"=w263:dbl, "Station 6 TCs.TC 18"=w262:dbl, "Station 6 TCs.TC 19"=w261:dbl, "Station 6 TCs.TC 20"=w260:dbl, "Station 6 TCs.TC 21"=w259:dbl, "Station 6 TCs.TC 22"=w258:dbl, "Station 6 TCs.TC 23"=w257:dbl, "Station 6 TCs.TC 24"=w256:dbl, "Station 6 TCs.TC 25"=w255:dbl, "Station 6 TCs.TC 26"=w254:dbl, "Station 6 TCs.TC 27"=w253:dbl, "Station 6 TCs.TC 28"=w252:dbl, "Station 6 TCs.TC 29"=w251:dbl, "Station 6 TCs.TC 30"=w250:dbl, "MX 5 (AUX Data).AUX 6_1"=w249:dbl, "MX 5 (AUX Data).AUX 6_2"=w248:dbl, "MX 5 (AUX Data).CAL CL6"=w247:dbl)
    }
    frame 7 {
      n9 = Unbundle By Name(w314) -> ("Station 7 TCs.TC 1"=w313:dbl, "Station 7 TCs.TC 2"=w312:dbl, "Station 7 TCs.TC 3"=w311:dbl, "Station 7 TCs.TC 4"=w310:dbl, "Station 7 TCs.TC 5"=w309:dbl, "Station 7 TCs.TC 6"=w308:dbl, "Station 7 TCs.TC 7"=w307:dbl, "Station 7 TCs.TC 8"=w306:dbl, "Station 7 TCs.TC 9"=w305:dbl, "Station 7 TCs.TC 10"=w304:dbl, "Station 7 TCs.TC 11"=w303:dbl, "Station 7 TCs.TC 12"=w302:dbl, "Station 7 TCs.TC 13"=w301:dbl, "Station 7 TCs.TC 14"=w300:dbl, "Station 7 TCs.TC 15"=w299:dbl, "Station 7 TCs.TC 16"=w298:dbl, "Station 7 TCs.TC 17"=w297:dbl, "Station 7 TCs.TC 18"=w296:dbl, "Station 7 TCs.TC 19"=w295:dbl, "Station 7 TCs.TC 20"=w294:dbl, "Station 7 TCs.TC 21"=w293:dbl, "Station 7 TCs.TC 22"=w292:dbl, "Station 7 TCs.TC 23"=w291:dbl, "Station 7 TCs.TC 24"=w290:dbl, "Station 7 TCs.TC 25"=w289:dbl, "Station 7 TCs.TC 26"=w288:dbl, "Station 7 TCs.TC 27"=w287:dbl, "Station 7 TCs.TC 28"=w286:dbl, "Station 7 TCs.TC 29"=w285:dbl, "Station 7 TCs.TC 30"=w284:dbl, "MX 5 (AUX Data).AUX 7_1"=w283:dbl, "MX 5 (AUX Data).AUX 7_2"=w282:dbl, "MX 5 (AUX Data).CAL CL7"=w281:dbl)
    }
    frame 8 {
      n10 = Unbundle By Name(w348) -> ("Station 8 TCs.TC 1"=w347:dbl, "Station 8 TCs.TC 2"=w346:dbl, "Station 8 TCs.TC 3"=w345:dbl, "Station 8 TCs.TC 4"=w344:dbl, "Station 8 TCs.TC 5"=w343:dbl, "Station 8 TCs.TC 6"=w342:dbl, "Station 8 TCs.TC 7"=w341:dbl, "Station 8 TCs.TC 8"=w340:dbl, "Station 8 TCs.TC 9"=w339:dbl, "Station 8 TCs.TC 10"=w338:dbl, "Station 8 TCs.TC 11"=w337:dbl, "Station 8 TCs.TC 12"=w336:dbl, "Station 8 TCs.TC 13"=w335:dbl, "Station 8 TCs.TC 14"=w334:dbl, "Station 8 TCs.TC 15"=w333:dbl, "Station 8 TCs.TC 16"=w332:dbl, "Station 8 TCs.TC 17"=w331:dbl, "Station 8 TCs.TC 18"=w330:dbl, "Station 8 TCs.TC 19"=w329:dbl, "Station 8 TCs.TC 20"=w328:dbl, "Station 8 TCs.TC 21"=w327:dbl, "Station 8 TCs.TC 22"=w326:dbl, "Station 8 TCs.TC 23"=w325:dbl, "Station 8 TCs.TC 24"=w324:dbl, "Station 8 TCs.TC 25"=w323:dbl, "Station 8 TCs.TC 26"=w322:dbl, "Station 8 TCs.TC 27"=w321:dbl, "Station 8 TCs.TC 28"=w320:dbl, "Station 8 TCs.TC 29"=w319:dbl, "Station 8 TCs.TC 30"=w318:dbl, "MX 5 (AUX Data).AUX 8_1"=w317:dbl, "MX 5 (AUX Data).AUX 8_2"=w316:dbl, "MX 5 (AUX Data).CAL CL8"=w315:dbl)
    }
  }
  n11 = Build Array(w44) -> (w37:dbl[])
  n12 = Build Array(w45) -> (w36:dbl[])
  n13 = Build Array(w46) -> (w35:dbl[])
  n14 = Build Array(w47) -> (w34:dbl[])
  n15 = Build Array(w48) -> (w33:dbl[])
  n16 = Build Array(w49) -> (w32:dbl[])
  n17 = Build Array(w50) -> (w31:dbl[])
  n18 = Build Array(w51) -> (w30:dbl[])
  n19 = Build Array(w52) -> (w29:dbl[])
  n20 = Build Array(w53) -> (w28:dbl[])
  n21 = Build Array(w54) -> (w27:dbl[])
  n22 = Build Array(w55) -> (w26:dbl[])
  n23 = Build Array(w56) -> (w25:dbl[])
  n24 = Build Array(w57) -> (w24:dbl[])
  n25 = Build Array(w58) -> (w23:dbl[])
  n26 = Build Array(w59) -> (w22:dbl[])
  n27 = Build Array(w60) -> (w21:dbl[])
  n28 = Build Array(w61) -> (w20:dbl[])
  n29 = Build Array(w62) -> (w19:dbl[])
  n30 = Build Array(w63) -> (w18:dbl[])
  n31 = Build Array(w64) -> (w17:dbl[])
  n32 = Build Array(w65) -> (w16:dbl[])
  n33 = Build Array(w66) -> (w15:dbl[])
  n34 = Build Array(w67) -> (w14:dbl[])
  n35 = Build Array(w68) -> (w13:dbl[])
  n36 = Build Array(w69) -> (w12:dbl[])
  n37 = Build Array(w70) -> (w11:dbl[])
  n38 = Build Array(w71) -> (w10:dbl[])
  n39 = Build Array(w72) -> (w9:dbl[])
  n40 = Build Array(w73) -> (w8:dbl[])
  n41 = Build Array(w74) -> (w7:dbl[])
  n42 = Build Array(w75) -> (w6:dbl[])
  n43 = Build Array(w76) -> (w5:dbl[])
  n44 = Build Array(w37, w36, w35, w34, w33, w32, w31, w30, w29, w28, w27, w26, w25, w24, w23, w22, w21, w20, w19, w18, w17, w16, w15, w14, w13, w12, w11, w10, w9, w8, w7, w6, w5) -> (w40:dbl[][])
  n45 = Index Array(array=w40, index (col)=0 ("disabled index (col)")) -> (element=w42:dbl[])  [unwired: 1 in]
  "Data MX (DBL)" <- w42
  n46 = call "UTILITY Double Array to String Array.vi"("Hex Array Out"=w42) -> ("Array"=w39:string[])  [unwired: 10 in]
  n47 = Build Array(w38, w39) -> (w2:string[][])
  n48 = Transpose 2D Array(2D array=w2) -> (transposed array=→"Data MX":string[][])
  "Error Out" <- "Error In"
  "Chamber 1 Data Out" <- "Chamber 1 Data in"
